vi "HTVacuumGUI.destructor.vi"(0 "i ref in":refnum<vi>, 5 "error in (no error)":errorcluster) -> (19 "error out":errorcluster)   [LabVIEW 2014, in "HTVacuumGUI.lvlib"]
doc: "This is the destructor of a class.\n\nLicense Agreement for this software:\n\nCopyright (C)\nGesellschaft für Schwerionenforschung, GSI\nPlanckstr. 1\n64291 Darmstadt\nGermany\n\nContact: D.Beck@gsi.de \n\nThis program is free software; you can redistribute it and/or modify it under the terms of the \nGNU General Public License as published by the Free Software Foundation; either version 2 of \nthe license, or (at your option) any later version.\n\nThis program is distributed in the hope that it will be useful, but WITHOUT ANY WARRANTY; \nwithout even the implied warranty of MERCHANTABILITY or FITNESS FOR A PARTICULAR PURPOSE. See the GNU General License for more details (http://www.gnu.org).\n\nGesellschaft für Schwerionenforschung, GSI\nPlanckstr. 1, 64291 Darmstadt, Germany\nFor all questions and ideas contact: M.Richter@gsi.de, H.Brand@gsi.de or D.Beck@gsi.de.\nLast update: 16-JUN-2004"
uses:
  HTVacuumGUI.lvlib
  CSCore/GUIs/GOGUserGUIs/DeviceBaseGUI/DeviceBaseGUI.lvlib
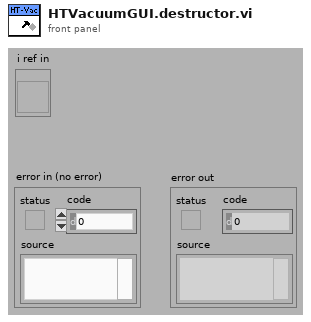
[diagram p1: front panel]
types:
  T1 = enum16{"SetAttribute", "GetAttribute", "CreateAttribute", "DestroyAttribute", "DestroyAllAtributes"}
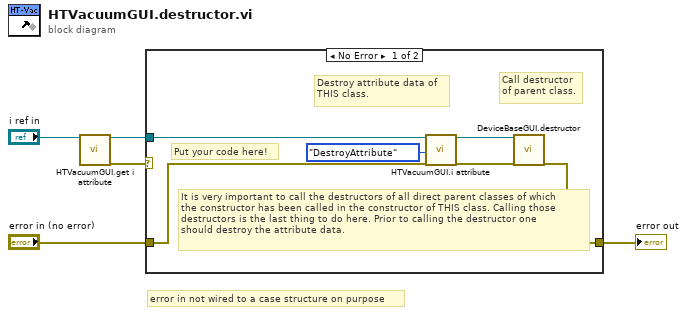
[diagram p0: block diagram]
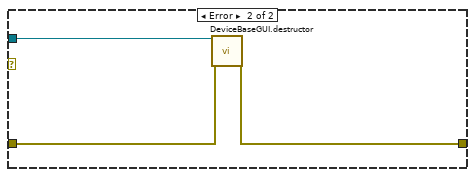
[diagram p2: hidden frame]
diagram:
  # "error in not wired to a case structure on purpose"
  n1 = call "HTVacuumGUI.get i attribute.vi"("i ref in"="i ref in") -> ("i ref out"=w2:refnum<vi>, "error out"=w1:errorcluster)  [unwired: 16 in, 1 out]
  n2 = case shown="No Error" w1 {
    tunnel: [w7 w13] -> w5
    tunnel: w2 -> [w10 w12]
    tunnel: "error in (no error)" -> [w9 w14]
    frame No Error {
      # "It is very important to call the destructors of all direct parent classes of which\nthe constructor has been called in the constructor of THIS class. Calling those\ndestructors is the last thing to do here. Prior to calling the destructor one \nshould destroy the attribute data."
      # "Put your code here!"
      # "Destroy attribute data of \nTHIS class."
      # "Call destructor\nof parent class."
      n3 = call "HTVacuumGUI.i attribute.vi"("VI Refnum"=w10, "Action"=T1."DestroyAttribute", "error in (no error)"=w9) -> ("VI Refnum out"=w6:refnum<vi>, "error out"=w8:errorcluster)  [unwired: 14 in, 1 out]
      n4 = call "DeviceBaseGUI.destructor.vi"("i ref in"=w6, "error in (no error)"=w8) -> ("error out"=w7:errorcluster)  [unwired: 17 in]
    }
    frame Error {
      n5 = call "DeviceBaseGUI.destructor.vi"("i ref in"=w12, "error in (no error)"=w14) -> ("error out"=w13:errorcluster)  [unwired: 17 in]
    }
  }
  "error out" <- w5
